vi "hysteresisCompensation2Polynoms.vi"(6 "PolynomBWD":dbl[](array[numeric])=[0.0, 1.0, 0.0, 0.0], 8 "error in (no error)":errorcluster, 9 "PolynomFWD":dbl[](array[numeric])=[0.0, 1.0, 0.0, 0.0], 10 "Uncorrected Shape":dbl[](array[numeric])) -> (0 "error out":errorcluster, 2 "Corrected Shape":dbl[](array[numeric]))   [LabVIEW 2016]
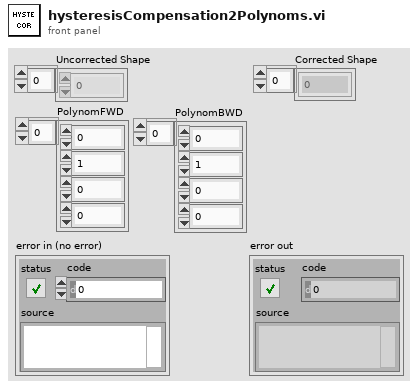
[diagram p1: front panel]
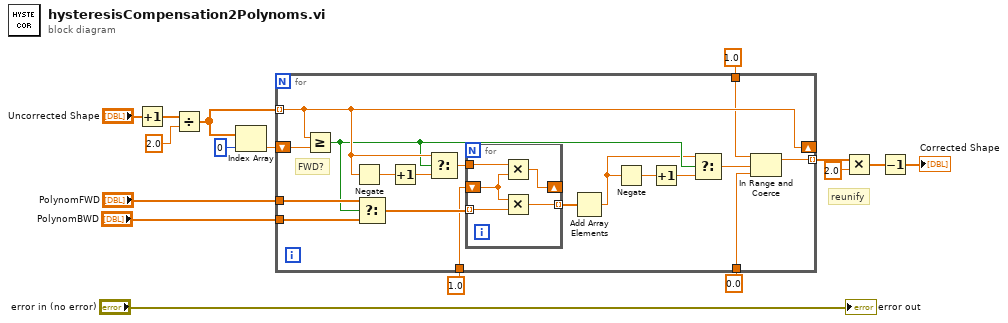
[diagram p0: block diagram]
diagram:
  # "reunify"
  n1 = Increment(x="Uncorrected Shape") -> (x+1=w3:dbl[])
  n2 = Divide(x=w3, y=2.0) -> (x/y=w8:dbl[])
  n3 = Index Array(array=w8, index=0) -> (element=w15:dbl)
  n4 = for {
    tunnel: w8 -> [w32] mode=indexing
    shift-right: [w32] -> _
    shift-left: w15 -> [w34]
    tunnel: "PolynomFWD" -> [w27]
    tunnel: [w31] -> w13 mode=indexing
    tunnel: 0.0 ("lower limit") -> [w30]
    tunnel: 1.0 ("upper limit") -> [w29]
    tunnel: "PolynomBWD" -> [w28]
    tunnel: 1.0 -> [w20]
    # "FWD?"
    n5 = Greater Or Equal?(x=w32, y=w34) -> (x >= y?=w25:bool)
    n6 = Negate(x=w32) -> (-x=w24:dbl)
    n7 = Select(t=w27, s=w25, f=w28) -> (s? t:f=w26:dbl[])
    n8 = Increment(x=w24) -> (x+1=w33:dbl)
    n9 = Select(t=w32, s=w25, f=w33) -> (s? t:f=w23:dbl)
    n10 = for {
      tunnel: w23 -> [w39]
      tunnel: w26 -> [w36] mode=indexing
      shift-right: [w38] -> _
      shift-left: w20 -> [w37]
      tunnel: [w35] -> w19 mode=indexing
      n11 = Multiply(x=w39, y=w37) -> (x*y=w38:dbl)
      n12 = Multiply(x=w37, y=w36) -> (x*y=w35:dbl)
    }
    n13 = Add Array Elements(numeric array=w19) -> (sum=w18:dbl)
    n14 = Negate(x=w18) -> (-x=w17:dbl)
    n15 = Increment(x=w17) -> (x+1=w21:dbl)
    n16 = Select(t=w18, s=w25, f=w21) -> (s? t:f=w22:dbl)
    n17 = In Range and Coerce(upper limit=w29, x=w22, lower limit=w30) -> (coerced(x)=w31:dbl)  [unwired: 1 out]
  }
  n18 = Multiply(x=w13, y=2.0) -> (x*y=w11:dbl[])
  n19 = Decrement(x=w11) -> (x-1=→"Corrected Shape":dbl[])
  "error out" <- "error in (no error)"
